vi "BM Stop.vi"(8 "error in (no error)":errorcluster, 11 "Bus Monitor in":refnum<class "Bus Monitor.lvclass">) -> (0 "error out":errorcluster, 3 "Bus Monitor out":refnum<class "Bus Monitor.lvclass">)   [LabVIEW 2020, in "Unit Tests.lvlib" / "Bus Monitor.lvclass"]
uses:
  Bus Monitor.lvclass
  Bus Monitor.lvclass/Bus Monitor.ctl
  <vilib>/addons/_JKI Toolkits/Caraya/classes/Assert/Assert True.vi
  1553 Session/1553 Session.lvclass
  Dependencies/FPGA Interface/FPGA Interface.lvclass
  <vilib>/addons/_JKI Toolkits/Caraya/classes/Test/Test.lvclass
  <vilib>/addons/_JKI Toolkits/Caraya/classes/Assert/Assert.lvclass
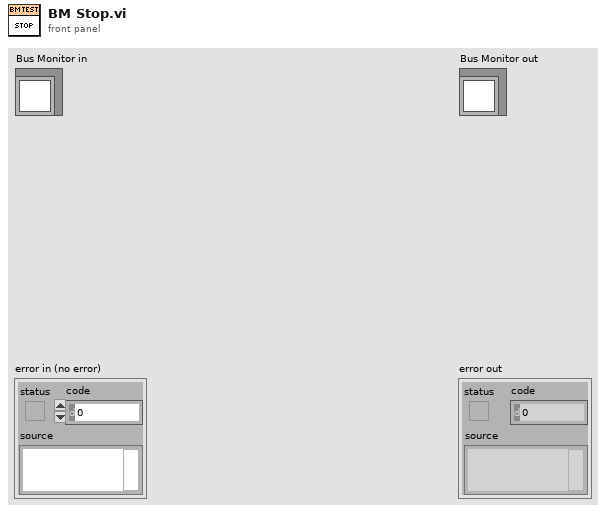
[diagram p1: front panel]
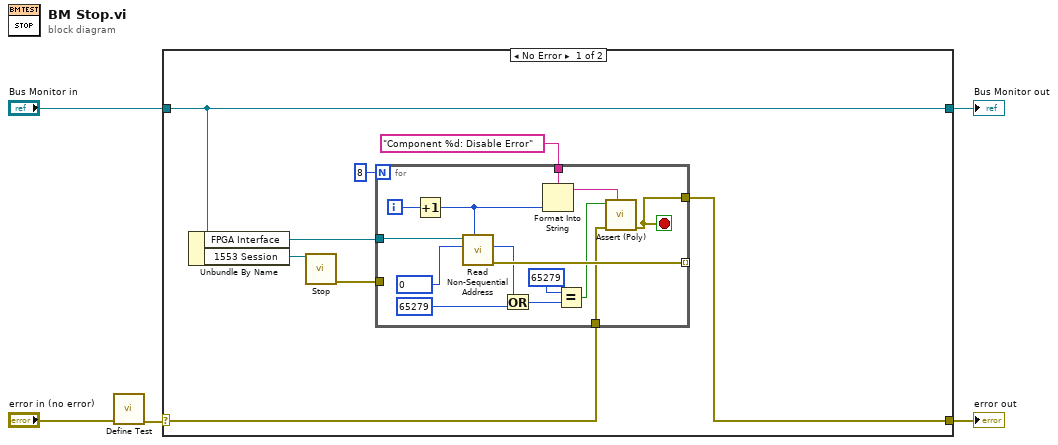
[diagram p0: block diagram]
diagram:
  n1 = call <vilib>:"Define Test.vi"("error in (no error)"="error in (no error)") -> ("error out"=w1:errorcluster)  [unwired: 9 in, 1 out]
  n2 = case shown="No Error" w1 {
    selector: w1 -> [w7 w29]
    tunnel: [w6 w29] -> w5
    tunnel: [w13 w28] -> w3
    tunnel: "Bus Monitor in" -> [w13 w28]
    frame No Error {
      n3 = Unbundle By Name(w13) -> ("FPGA Interface"=w11:refnum<class "FPGA Interface.lvclass">, "1553 Session"=w12:refnum<class "1553 Session.lvclass">)
      n4 = call-dynamic "Stop.vi"("1553 Board in"=w12) -> ("error out"=w10:errorcluster)  [unwired: 9 in, 1 out]
      n5 = for {
        N: 8 -> [_]
        tunnel: w11 -> [w27]
        tunnel: "Component %d: Disable Error" ("custom report message (\"\")") -> [w24]
        tunnel: w7 -> [w15]
        tunnel: [w17] -> w6
        tunnel: [w22] -> _ mode=indexing
        tunnel: w10 -> [_]
        i -> [w26]
        stop <- w17 stop-if-true
        n6 = Increment(x=w26) -> (x+1=w23:i32)
        n7 = call-dynamic "Read Non-Sequential Address.vi"("Target IC (1-8)"=w23, "Address"=u16 0, "FPGA Interface in"=w27) -> ("error out"=w22:errorcluster, "Data"=w19:u16)  [unwired: 7 in]
        n8 = Or(x=w19, y=u16 65279) -> (x .or. y?=w20:u16)
        n9 = Format Into String(format string=w24, w23) -> (resulting string=w14:string)  [unwired: 2 in, 1 out]
        n10 = Equal?(x=u16 65279, y=w20) -> (x = y?=w16:bool)
        n11 = call-poly <vilib>:"Assert (Poly).vi"("Label"=w14, "error in (no error)"=w15, "True?"=w16) -> ("error out"=w17:errorcluster)  [unwired: 7 in, 1 out]
      }
    }
    frame Error {
    }
  }
  "error out" <- w5
  "Bus Monitor out" <- w3
